vi "F Dwf Digital In Trigger Position Get.vi"(8 "error in (no error)":errorcluster, 10 "pcSamplesAfterTrigger":u32, 11 "hdwf":i32) -> (0 "error out":errorcluster, 2 "pcSamplesAfterTrigger out":u32, 3 "function return":i32)   [LabVIEW 2019, in "Olasdwf.lvlib"]
doc: "DWFAPI int FDwfDigitalInTriggerPositionGet(HDWF hdwf, unsigned int *pcSamplesAfterTrigger);"
uses:
  Olasdwf.lvlib
  Windows/System32/dwf.dll
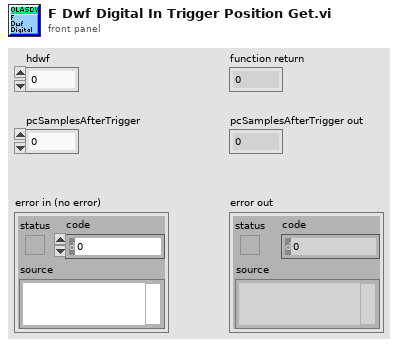
[diagram p1: front panel]
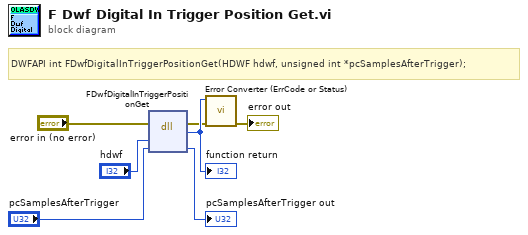
[diagram p0: block diagram]
diagram:
  # "DWFAPI int FDwfDigitalInTriggerPositionGet(HDWF hdwf, unsigned int *pcSamplesAfterTrigger);"
  n1 = dll-call lib="C:/Windows/System32/dwf.*" fn="FDwfDigitalInTriggerPositionGet"(error in="error in (no error)", "hdwf"="hdwf", "pcSamplesAfterTrigger"="pcSamplesAfterTrigger") -> (error out=w2:errorcluster, w7:i32, "pcSamplesAfterTrigger"=→"pcSamplesAfterTrigger out":u32)  [unwired: 3 in, 1 out]
  "function return" <- w7
  n2 = call "Error Converter (ErrCode or Status).vi"("error in (no error)"=w2, "error code"=w7) -> ("error out"=→"error out":errorcluster)  [unwired: 9 in]
